vi "Read Parent State.vi"(8 "error in (no error)":errorcluster, 11 "State Machine Actor in":refnum<class "State Machine Actor.lvclass">) -> (0 "error out":errorcluster, 2 "Parent State":refnum<class "_State Machine Actor.lvclass">, 3 "State Machine Actor out":refnum<class "State Machine Actor.lvclass">)   [LabVIEW 2024, in "State Machine Actor.lvlib" / "State Machine Actor.lvclass"]
uses:
  State Machine Actor.lvclass
  State Machine Actor.lvclass/State Machine Actor.ctl
  _State Machine Actor/_State Machine Actor/_State Machine Actor.lvclass
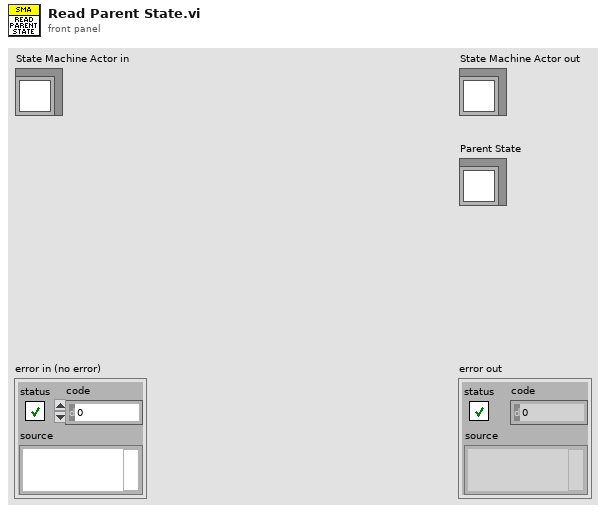
[diagram p1: front panel]
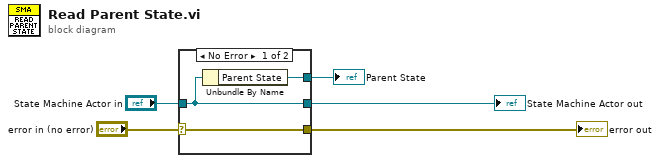
[diagram p0: block diagram]
diagram:
  n1 = case shown="No Error" "error in (no error)" {
    selector: "error in (no error)" -> [w8 w9]
    tunnel: [w8 w9] -> w4
    tunnel: [w7 w10] -> w2
    tunnel: "State Machine Actor in" -> [w7 w10]
    tunnel: [w6 _] -> w1
    frame No Error {
      n2 = Unbundle By Name(w7) -> ("Parent State"=w6:refnum<class "_State Machine Actor.lvclass">)
    }
    frame Error {
    }
  }
  "error out" <- w4
  "State Machine Actor out" <- w2
  "Parent State" <- w1
